vi "Sort_Dust_Array.vi"(1 "Descending?":bool, 2 "Order by...":T1(ring), 3 "Array In":T2[](array[typedef])) -> (0 "Array out":T2[](array[typedef]))   [LabVIEW 2013]
uses:
  dust_list.ctl
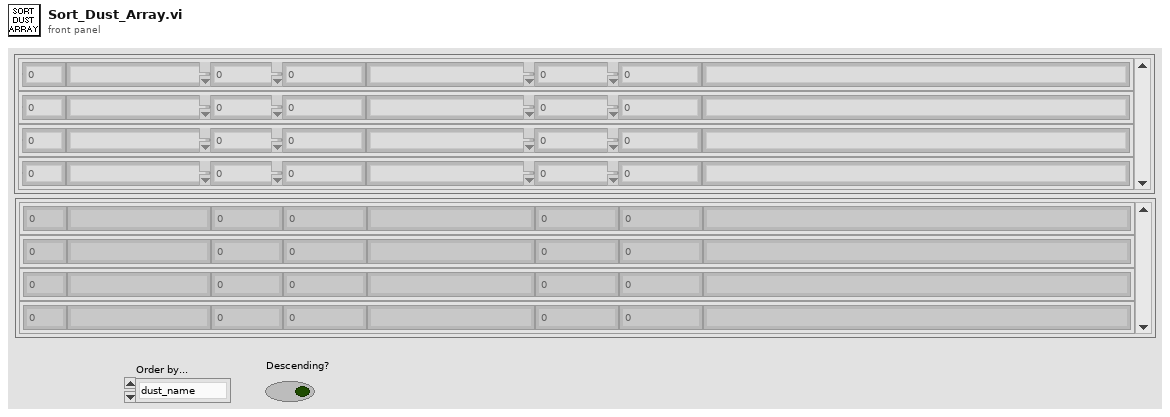
[diagram p1: front panel]
types:
  T1 = enum16{"dust_name", "dust_density", "source_weight", "bottle_weight", "dust_weight"}
  T2 = typedef "dust_list.ctl" = cluster{"id_dust_type":i32, "dust_name":string, "dust_density":dbl, "source_weight":dbl, "size":string, "bottle_weight":dbl, "dust_mass":dbl, "comments":string}
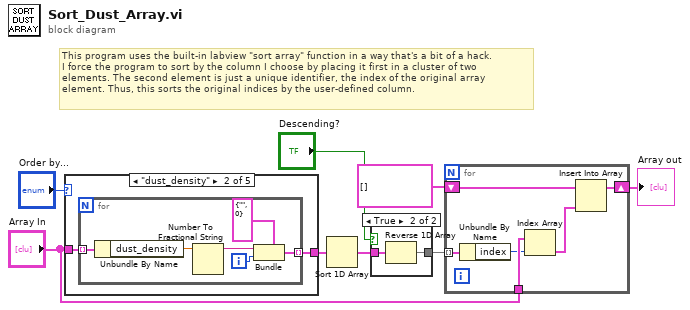
[diagram p0: block diagram]
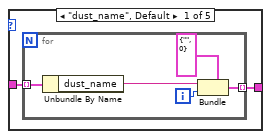
[diagram p3: hidden frame]
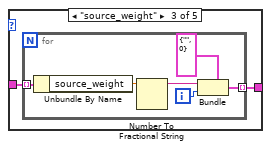
[diagram p4: hidden frame]
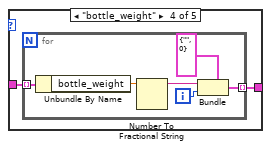
[diagram p5: hidden frame]
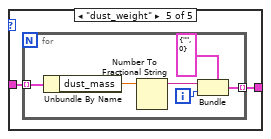
[diagram p6: hidden frame]
diagram:
  # "This program uses the built-in labview \"sort array\" function in a way that's a bit of a hack.\nI force the program to sort by the column I choose by placing it first in a cluster of two\nelements. The second element is just a unique identifier, the index of the original array\nelement. Thus, this sorts the original indices by the user-defined column."
  n1 = case shown="\"dust_density\"" "Order by..." {
    tunnel: "Array In" -> [w10 w17 w25 w33 w41]
    tunnel: [w9 w16 w24 w32 w40] -> w7
    frame "dust_name", Default {
      n2 = for {
        tunnel: w10 -> [w15] mode=indexing
        tunnel: [w13] -> w9 mode=indexing
        i -> [w12]
        n3 = Unbundle By Name(w15) -> ("dust_name"=w14:string)
        n4 = Bundle(cluster=cluster{"dust_name":string, "index":i32} {"dust_name"="", "index"=0}, "dust_name"=w14, "index"=w12) -> (w13:cluster{"dust_name":string, "index":i32})
      }
    }
    frame "dust_density" {
      n5 = for {
        tunnel: w17 -> [w23] mode=indexing
        tunnel: [w21] -> w16 mode=indexing
        i -> [w20]
        n6 = Unbundle By Name(w23) -> ("dust_density"=w22:dbl)
        n7 = Number To Fractional String(number=w22) -> (F-format string=w18:string)  [unwired: 3 in]
        n8 = Bundle(cluster=cluster{"dust_name":string, "index":i32} {"dust_name"="", "index"=0}, "dust_name"=w18, "index"=w20) -> (w21:cluster{"dust_name":string, "index":i32})
      }
    }
    frame "source_weight" {
      n9 = for {
        tunnel: w25 -> [w31] mode=indexing
        tunnel: [w29] -> w24 mode=indexing
        i -> [w28]
        n10 = Unbundle By Name(w31) -> ("source_weight"=w30:dbl)
        n11 = Number To Fractional String(number=w30) -> (F-format string=w26:string)  [unwired: 3 in]
        n12 = Bundle(cluster=cluster{"dust_name":string, "index":i32} {"dust_name"="", "index"=0}, "dust_name"=w26, "index"=w28) -> (w29:cluster{"dust_name":string, "index":i32})
      }
    }
    frame "bottle_weight" {
      n13 = for {
        tunnel: w33 -> [w39] mode=indexing
        tunnel: [w37] -> w32 mode=indexing
        i -> [w36]
        n14 = Unbundle By Name(w39) -> ("bottle_weight"=w38:dbl)
        n15 = Number To Fractional String(number=w38) -> (F-format string=w34:string)  [unwired: 3 in]
        n16 = Bundle(cluster=cluster{"dust_name":string, "index":i32} {"dust_name"="", "index"=0}, "dust_name"=w34, "index"=w36) -> (w37:cluster{"dust_name":string, "index":i32})
      }
    }
    frame "dust_weight" {
      n17 = for {
        tunnel: w41 -> [w47] mode=indexing
        tunnel: [w45] -> w40 mode=indexing
        i -> [w44]
        n18 = Unbundle By Name(w47) -> ("dust_mass"=w46:dbl)
        n19 = Number To Fractional String(number=w46) -> (F-format string=w42:string)  [unwired: 3 in]
        n20 = Bundle(cluster=cluster{"dust_name":string, "index":i32} {"dust_name"="", "index"=0}, "dust_name"=w42, "index"=w44) -> (w45:cluster{"dust_name":string, "index":i32})
      }
    }
  }
  n21 = Sort 1D Array(array=w7) -> (sorted array=w5:cluster{"dust_name":string, "index":i32}[])
  n22 = case shown="True" "Descending?" {
    tunnel: w5 -> [w48 w50]
    tunnel: [w48 w49] -> w4
    frame False {
    }
    frame True {
      n23 = Reverse 1D Array(array=w50) -> (reversed array=w49:cluster{"dust_name":string, "index":i32}[])
    }
  }
  n24 = for {
    tunnel: w4 -> [w56] mode=indexing
    shift-right: [w54] -> w1
    shift-left: T2[] [] ("Array In") -> [w55]
    tunnel: "Array In" -> [w53]
    n25 = Unbundle By Name(w56) -> ("index"=w51:i32)
    n26 = Index Array(array=w53, index=w51) -> (element=w52:T2)
    n27 = Insert Into Array(array=w55, new element=w52) -> (w54:T2[])  [unwired: 1 in]
  }
  "Array out" <- w1
